vi "pp2_trial_Select.vi"(0 "Trial Types":T4[](array[typedef])=[{"Trial Type Number"=1, "Trial Type"=enum."GO", "Trial Weight"=1, "Shock (mA)"=-1.0, "Duration (ms)"=250.0, "Sound Type"=enum."04 FM Sweep", "Stim P1"=4000.0, "Stim P2"=0.0, "Stim P3"=0.0, "Stim P4"=2000.0}, {"Trial Type Number"=2, "Trial Type"=enum."NOGO", "Trial Weight"=1, "Shock (mA)"=-1.0, "Duration (ms)"=250.0, "Sound Type"=enum."04 FM Sweep", "Stim P1"=2000.0, "Stim P2"=0.0, "Stim P3"=0.0, "Stim P4"=4000.0}] {"Shock (mA)" min=-1.0 max=5.0; "Trial Weight" step=1; "Duration (ms)" min=0.0 max=1.0; "Trial Type Number" min=1 step=1}, 5 "Code":i32) -> (4 "Cluster":T1={"Trial Type Number"=1, "Trial Type"=enum."GO", "Trial Weight"=100, "Shock (mA)"=0.3, "Duration (ms)"=0.25, "Sound Type"=enum."04 FM Sweep", "Stim P1"=2000.0, "Stim P2"=4000.0, "Stim P3"=0.0, "Stim P4"=0.0} {"Shock (mA)" min=-1.0 max=5.0; "Trial Weight" step=1; "Duration (ms)" min=0.0 max=1.0; "Trial Type Number" min=1 max=256 step=1})   [LabVIEW 2013]
doc: "This VI loads the next trial into \"current loaded trial\" in the State info, and applies approrpiate variable shock if applicable"
uses:
  pp2_Trial.ctl
  pp2_CTL_TrialType.ctl
  labolabo2/waveforms/WFTypes.ctl
  pp2_CTL_Trial.ctl
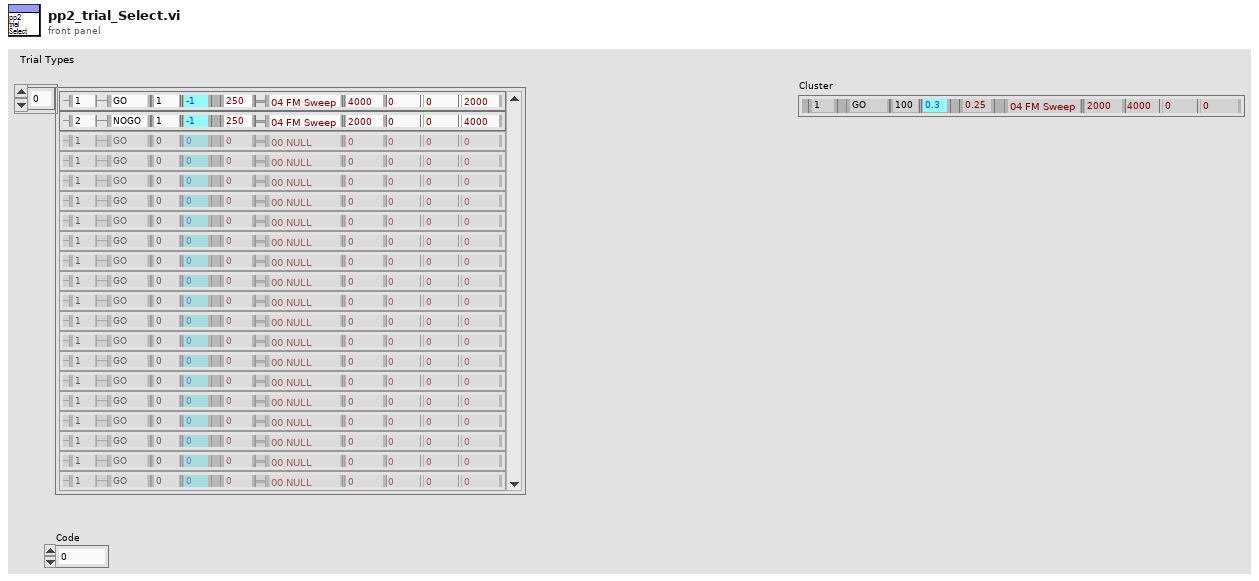
[diagram p1: front panel]
types:
  T1 = typedef "pp2_CTL_Trial.ctl" = cluster{"Trial Type Number":i16, "Trial Type":T2, "Trial Weight":u32, "Shock (mA)":dbl, "Duration (ms)":dbl, "Sound Type":T3, "Stim P1":dbl, "Stim P2":dbl, "Stim P3":dbl, "Stim P4":dbl}
  T2 = typedef "pp2_CTL_TrialType.ctl" = enum16{"OFF", "GO", "NOGO", "TEST"}
  T3 = typedef "WFTypes.ctl" = enum16{"00 NULL", "01 DC", "02 Noise", "03 Pure Tone", "04 FM Sweep"}
  T4 = typedef "pp2_Trial.ctl" = cluster{"Trial Type Number":u8, "Trial Type":T2, "Trial Weight":u32, "Shock (mA)":dbl, "Duration (ms)":dbl, "Sound Type":T3, "Stim P1":dbl, "Stim P2":dbl, "Stim P3":dbl, "Stim P4":dbl}
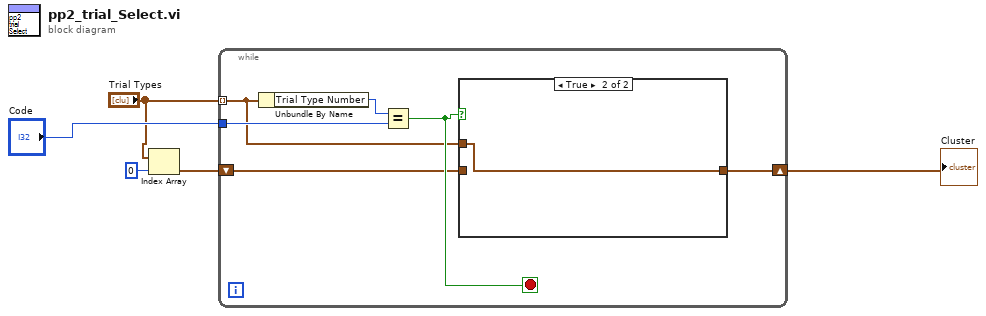
[diagram p0: block diagram]
diagram:
  n1 = Index Array(array="Trial Types", index=0) -> (element=w2:T4)
  n2 = while {
    tunnel: "Trial Types" -> [w8] mode=indexing
    tunnel: "Code" -> [w10]
    shift-right: [w6] -> w1
    shift-left: w2 -> [w7]
    stop <- w9 stop-if-true
    n3 = Unbundle By Name(w8) -> ("Trial Type Number"=w11:u8)
    n4 = Equal?(x=w11, y=w10) -> (x = y?=w9:bool)
    n5 = case shown="True" w9 {
      tunnel: w8 -> [_ w13]
      tunnel: w7 -> [w12 _]
      tunnel: [w12 w13] -> w6
      frame False {
      }
      frame True {
      }
    }
  }
  "Cluster" <- w1
